vi "ReadFromDAQSingleChunk.vi"() -> ()   [LabVIEW 2025]
uses:
  <vilib>/DAQmx/read.llb/DAQmx Read (Analog 1D Wfm NChan NSamp).vi
  <vilib>/DAQmx/create/channels.llb/DAQmx Create Channel (AI-Voltage-Basic).vi
  <vilib>/DAQmx/configure/timing.llb/DAQmx Timing (Sample Clock).vi
  <vilib>/DAQmx/miscellaneous.llb/DAQmx Fill In Error Info.vi
panel:
  out "data":waveform(dbl)[](array[waveform])
  out "error out":errorcluster
  out "Waveform Graph":waveform(dbl)[](graph)
  in  "error in":errorcluster
  in  "channel settings":T1={"max value"=5.0, "min value"=-5.0, "physical channels"="Dev1/ai2", "input terminal configuration"=-1, "units"=10348} {"input terminal configuration" items=["Default"=-1, "RSE"=10083, "NRSE"=10078, "Differential"=10106, "Pseudodifferential"=12529]; "units" items=["Volts"=10348, "From Custom Scale"=10065]}
  in  "clock settings":T2={"sample mode"=10178, "samples per channel"=1000, "rate"=1000.0} {"sample mode" items=["Finite Samples"=10178, "Continuous Samples"=10123, "Hardware Timed Single Point"=12522]}
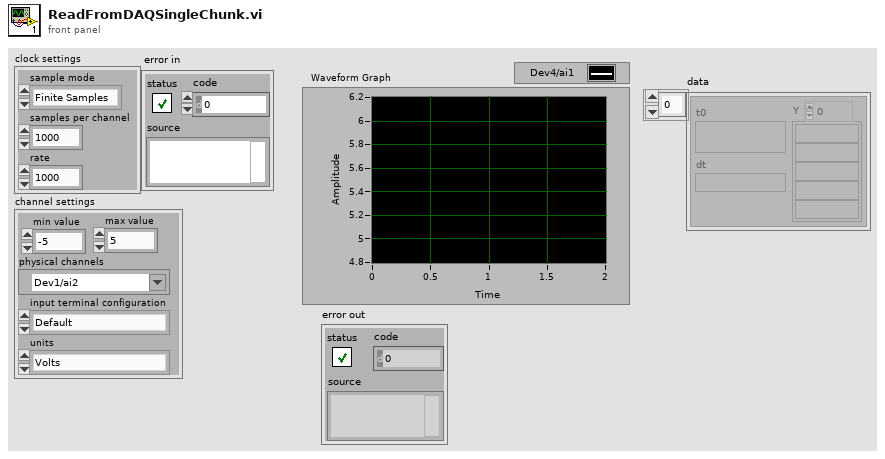
[diagram p1: front panel]
types:
  T1 = cluster{"max value":dbl, "min value":dbl, "physical channels":tag, "input terminal configuration":i32, "units":i32}
  T2 = cluster{"sample mode":i32, "samples per channel":i32, "rate":dbl}
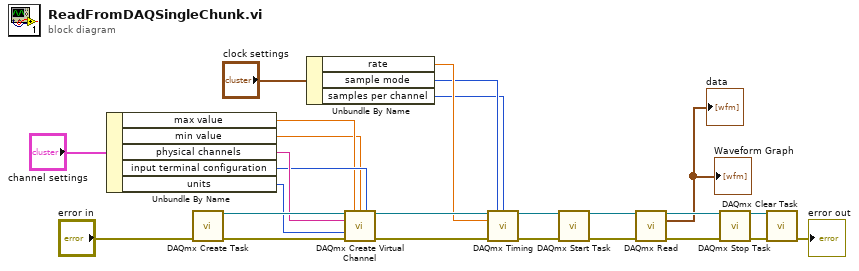
[diagram p0: block diagram]
diagram:
  n1 = Unbundle By Name("channel settings") -> ("max value"=w5:dbl, "min value"=w4:dbl, "physical channels"=w8:tag, "input terminal configuration"=w7:i32, "units"=w6:i32)
  n2 = call <vilib>:"DAQmx Create Task.vi"("error in"="error in") -> ("task out"=w24:refnum<k21>, "error out"=w23:errorcluster)  [unwired: 13 in]
  n3 = Unbundle By Name("clock settings") -> ("rate"=w11:dbl, "sample mode"=w10:i32, "samples per channel"=w9:i32)
  n4 = call-poly <vilib>:"DAQmx Create Virtual Channel.vi"("task in"=w24, "maximum value"=w5, "minimum value"=w4, "input terminal configuration"=w7, "physical channels"=w8, "units"=w6, "error in"=w23) -> ("task out"=w25:refnum<k21>, "error out"=w22:errorcluster)  [unwired: 7 in]
  n5 = call-poly <vilib>:"DAQmx Timing.vi"("task/channels in"=w25, "sample mode"=w10, "samples per channel"=w9, "rate"=w11, "error in"=w22) -> ("task out"=w21:refnum<k21>, "error out"=w20:errorcluster)  [unwired: 9 in]
  n6 = call <vilib>:"DAQmx Start Task.vi"("task/channels in"=w21, "error in"=w20) -> ("task out"=w19:refnum<k21>, "error out"=w18:errorcluster)  [unwired: 12 in]
  n7 = call-poly <vilib>:"DAQmx Read.vi"("task/channels in"=w19, "error in"=w18) -> ("task out"=w17:refnum<k21>, "data"=→"Waveform Graph" →"data":waveform(dbl)[], "error out"=w16:errorcluster)  [unwired: 11 in]
  n8 = call <vilib>:"DAQmx Stop Task.vi"("task/channels in"=w17, "error in"=w16) -> ("task out"=w15:refnum<k21>, "error out"=w14:errorcluster)  [unwired: 12 in]
  n9 = call <vilib>:"DAQmx Clear Task.vi"("task in"=w15, "error in"=w14) -> ("error out"=→"error out":errorcluster)  [unwired: 13 in]
